vi "TDMS.CheckFileProperties.vi"(8 "error in (no error)":errorcluster, 11 "Data":path) -> (0 "error out":errorcluster, 3 "Found All":bool)   [LabVIEW 2015, in "NIAnalysis.lvlib"]
uses:
  NIAnalysis.lvlib
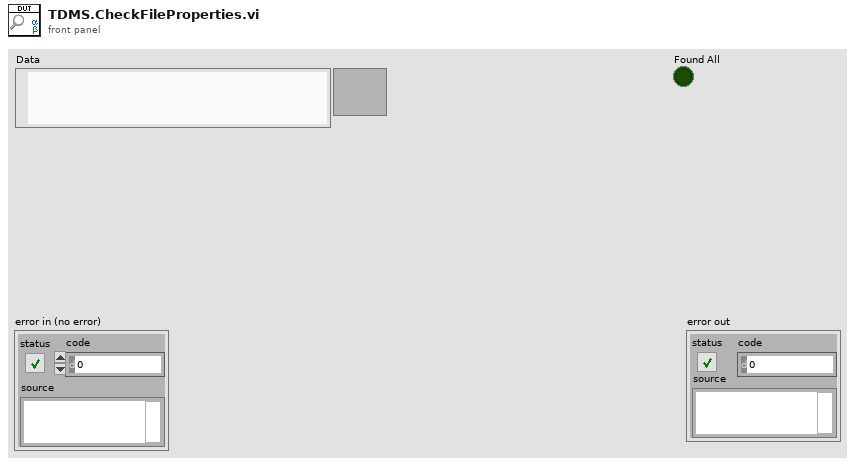
[diagram p1: front panel]
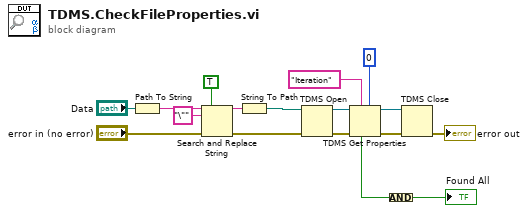
[diagram p0: block diagram]
diagram:
  n1 = Path To String(path="Data") -> (string=w7:string)
  n2 = Search and Replace String(replace all?=TRUE ("replace all? (F)"), input string=w7, search string="\"", error in="error in (no error)") -> (result string=w8:string, error out=w2:errorcluster)  [unwired: 4 in, 2 out]
  n3 = String To Path(string=w8) -> (path=w1:path)
  n4 = TDMS Open(8:w2, 11:w1) -> (0:w15:errorcluster, 3:w16:refnum<k34>)  [unwired: 5 in]
  n5 = TDMS Get Properties(5:0 ("Iteration"), 7:"Iteration" ("property name"), 8:w15, 11:w16) -> (0:w11:errorcluster, 3:w10:refnum<k34>, 6:w13:bool)  [unwired: 2 in, 3 out]
  n6 = Compound Arithmetic op=AND(w13) -> (→"Found All":bool)
  n7 = TDMS Close(8:w11, 11:w10) -> (0:→"error out":errorcluster)  [unwired: 1 out]
